vi "Autonomous camera.vi"() -> ()   [LabVIEW 2013]
doc: "This VI is called when autonomous begins, and will automatically be terminated when autonomous ends. You can carry out timed or sensor driven robot movement independently without needing to return to the caller."
uses:
  2014 Target Detection/TargetType.ctl
  Robot Global Data.vi
panel:
  in  "Not hot":i32
  out "Goal State":T1
  in  "Down break":dbl=20.0 format="%#_13g"
  in  "Hot":i32=50
  in  "Move":i32=275
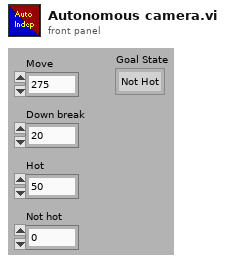
[diagram p1: front panel]
types:
  T1 = typedef "TargetType.ctl" = enum16{"Not Hot", "Hot"}
  T2 = cluster{"Scores":cluster{"Total":dbl, "Left":dbl, "Right":dbl, "Ratio":dbl, "Vertical":dbl, "index":i32, "State":T1}, "Verticals":cluster{"Horizontal?":bool, "Aspect Score":dbl, "Rect Score":dbl, cluster{"Left":dbl, "Top":dbl, "Right":dbl, "Bottom":dbl}, "Equiv H":dbl, "Equiv V":dbl}, "Horizontals":cluster{"Horizontal?":bool, "Aspect Score":dbl, "Rect Score":dbl, cluster{"Left":dbl, "Top":dbl, "Right":dbl, "Bottom":dbl}, "Equiv H":dbl, "Equiv V":dbl}, "Distance ft":dbl, "Center":cluster{"X":dbl, "Y":dbl}}[]
  T3 = cluster{"Scores":cluster{"Total":dbl, "Left":dbl, "Right":dbl, "Ratio":dbl, "Vertical":dbl, "index":i32, "State":T1}, "Verticals":cluster{"Horizontal?":bool, "Aspect Score":dbl, "Rect Score":dbl, cluster{"Left":dbl, "Top":dbl, "Right":dbl, "Bottom":dbl}, "Equiv H":dbl, "Equiv V":dbl}, "Horizontals":cluster{"Horizontal?":bool, "Aspect Score":dbl, "Rect Score":dbl, cluster{"Left":dbl, "Top":dbl, "Right":dbl, "Bottom":dbl}, "Equiv H":dbl, "Equiv V":dbl}, "Distance ft":dbl, "Center":cluster{"X":dbl, "Y":dbl}}
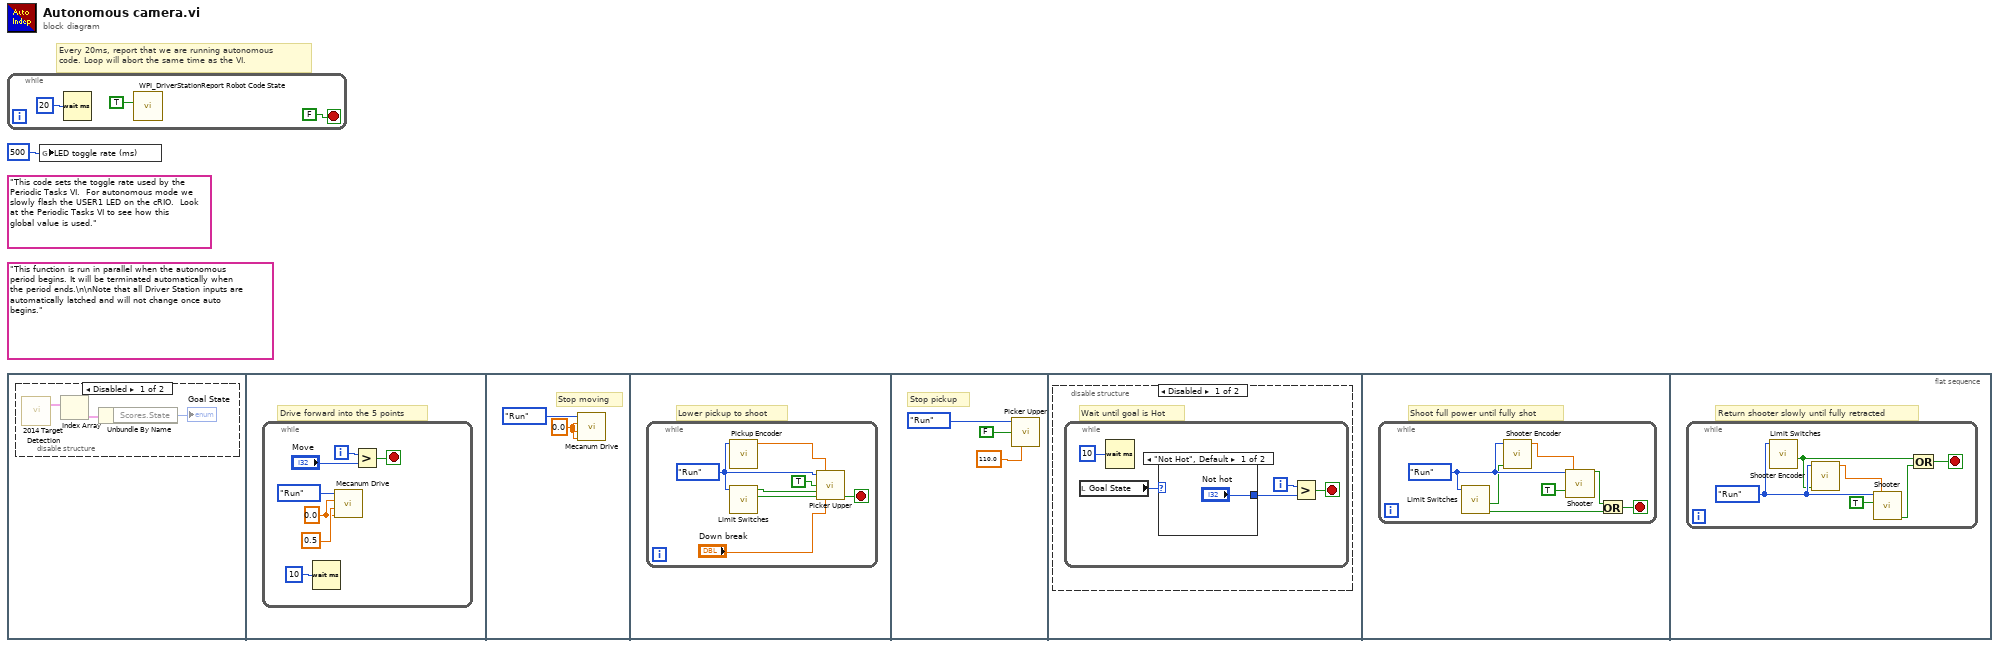
[diagram p0: block diagram]
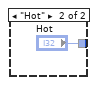
[diagram p3: hidden frame]
diagram:
  (unwired) "This function is run in parallel when the autonomous period begins. It will be terminated automatically when the period ends.\n\nNote that all Driver Station inputs are automatically latched and will not change once auto begins."
  (unwired) "This code sets the toggle rate used by the Periodic Tasks VI.  For autonomous mode we slowly flash the USER1 LED on the cRIO.  Look at the Periodic Tasks VI to see how this global value is used."
  # "Every 20ms, report that we are running autonomous\ncode. Loop will abort the same time as the VI."
  n1 = while {
    stop <- FALSE stop-if-true
    n2 = Wait (ms)(milliseconds to wait=u32 20) -> ()  [unwired: 1 out]
    n3 = call <vilib>:"WPI_DriverStationReport Robot Code State.vi"("Autonomous"=TRUE) -> ()  [unwired: 10 in, 1 out]
  }
  n4 = flat-sequence {
    frame #0 {
      n5 = disable-structure shown="Disabled" {
        frame Disabled {
          n6 = call "2014 Target Detection.vi"() -> ("Target Info"=w7:T2)  [unwired: 1 in, 1 out]
          n7 = Index Array(array=w7) -> (element=w6:T3)  [unwired: 1 in]
          n8 = Unbundle By Name(w6) -> ("Scores.State"=→"Goal State":T1)
        }
        frame Enabled {
        }
      }
    }
    frame #1 {
      # "Drive forward into the 5 points"
      n9 = while {
        i -> [w14]
        stop <- w9 stop-if-true
        w8 = 0.0 ("Strafing")
        n10 = Wait (ms)(milliseconds to wait=u32 10) -> ()  [unwired: 1 out]
        n11 = call "Mecanum Drive.vi"("Turn"=w8, "Forward/Backward"=0.5 ("F/R"), "Strafe"=w8, "State Control"=enum16{"Open", "Run", "End"}."Run") -> ()  [unwired: 4 in]
        n12 = Greater?(x=w14, y="Move") -> (0:w9:bool)
      }
    }
    frame #2 {
      w15 = 0.0 ("F/R")
      # "Stop moving"
      n13 = call "Mecanum Drive.vi"("Turn"=w15, "Forward/Backward"=w15, "Strafe"=w15, "State Control"=enum16{"Open", "Run", "End"}."Run") -> ()  [unwired: 4 in]
    }
    frame #3 {
      # "Lower pickup to shoot"
      n14 = while {
        stop <- w23 stop-if-true
        w21 = enum16{"Open", "Run", "End"}."Run" ("State Control")
        n15 = call "Pickup Encoder.vi"("State Control"=w21) -> ("Encoder Degrees"=w20:dbl)  [unwired: 3 in, 3 out]
        n16 = call "Limit Switches.vi"("State Control"=w21) -> ("Picker Upper Bottom"=w22:bool, "Picker Upper Top"=w18:bool)  [unwired: 7 in, 2 out]
        n17 = call "Picker Upper.vi"("State Control"=w21, "Encoder"=w20, "Down"=TRUE, "Top limit"=w18, "Bottom Limit"=w22, "Down break"="Down break") -> ("Fully down?"=w23:bool)  [unwired: 8 in, 1 out]
      }
    }
    frame #4 {
      # "Stop pickup"
      n18 = call "Picker Upper.vi"("State Control"=enum16{"Open", "Run", "End"}."Run", "Down"=FALSE, "Down break"=110.0) -> ()  [unwired: 11 in, 2 out]
    }
    frame #5 {
      n19 = disable-structure shown="Disabled" {
        frame Disabled {
          # "Wait until goal is Hot"
          n20 = while {
            i -> [w31]
            stop <- w30 stop-if-true
            n21 = local read "Goal State"() -> (w28:T1)
            n22 = Wait (ms)(milliseconds to wait=u32 10) -> ()  [unwired: 1 out]
            n23 = case shown="\"Not Hot\", Default" w28 {
              tunnel: ["Not hot" "Hot"] -> w27
              frame "Not Hot", Default {
              }
              frame "Hot" {
              }
            }
            n24 = Greater?(x=w31, y=w27) -> (0:w30:bool)
          }
        }
        frame Enabled {
        }
      }
    }
    frame #6 {
      # "Shoot full power until fully shot"
      n25 = while {
        stop <- w37 stop-if-true
        w40 = enum16{"Open", "Run", "End"}."Run" ("State Control")
        n26 = call "Limit Switches.vi"("State Control"=w40) -> ("Shooter Top"=w38:bool, "Shooter Bottom"=w35:bool)  [unwired: 7 in, 2 out]
        n27 = call "Shooter Encoder.vi"("Reset Encoder?"=w35, "State Control"=w40) -> ("Encoder Degrees"=w36:dbl)  [unwired: 2 in, 3 out]
        n28 = call "Shooter.vi"("State Control"=w40, "4 ft"=TRUE, "Encoder"=w36) -> ("Fully shot?"=w39:bool)  [unwired: 15 in, 1 out]
        n29 = Or(x=w39, y=w38) -> (x .or. y?=w37:bool)
      }
    }
    frame #7 {
      # "Return shooter slowly until fully retracted"
      n30 = while {
        stop <- w43 stop-if-true
        w46 = enum16{"Open", "Run", "End"}."Run" ("State Control")
        n31 = call "Limit Switches.vi"("State Control"=w46) -> ("Shooter Bottom"=w42:bool)  [unwired: 7 in, 3 out]
        n32 = call "Shooter Encoder.vi"("Reset Encoder?"=w42, "State Control"=w46) -> ("Encoder Degrees"=w45:dbl)  [unwired: 2 in, 3 out]
        n33 = call "Shooter.vi"("State Control"=w46, "Return"=TRUE, "Encoder"=w45) -> ("Fully retracted?"=w44:bool)  [unwired: 15 in, 1 out]
        n34 = Or(x=w42, y=w44) -> (x .or. y?=w43:bool)
      }
    }
  }
  n35 = global write "Robot Global Data.vi" "LED toggle rate (ms)"(u32 500 ("LED ms toggle rate")) -> ()
